vi "Cleanup.vi"(8 "error in":errorcluster, 11 "Refnum In":refnum<vi>) -> (0 "error out":errorcluster, 3 "Refnum Out":refnum<vi>)   [LabVIEW 2020]
doc: "Initializes the library with a serial comport as the transport method"
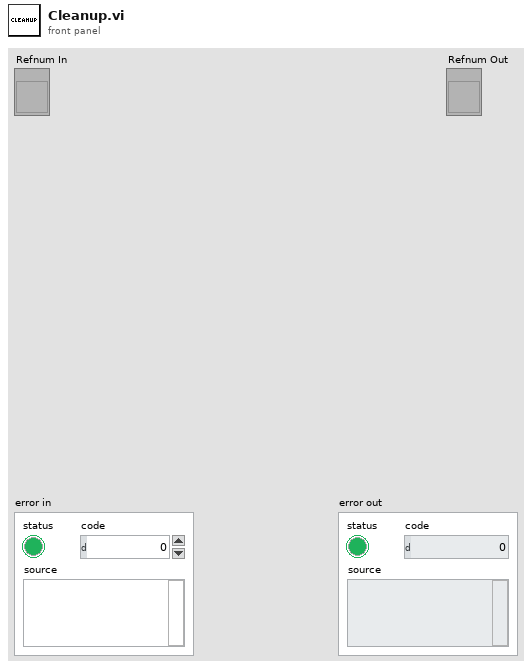
[diagram p1: front panel]
types:
  T1 = typedef "ConnectionParameters.ctl" = cluster{"Serial Communication":cluster{"Comport":refnum<visa-resource-name>, "No Response Timeout Ms":u32, "Response Complete Timeout Ms":u32, "Max Rx Length":u32, "Baud Rate":u32}, "Selected Transport":T2, "Initializer File Path":path, "Cleaner File Path":path, "Transporter File Path":path}
  T2 = typedef "SupportedTransports.ctl" = enum16{"Serial Communication Port"}
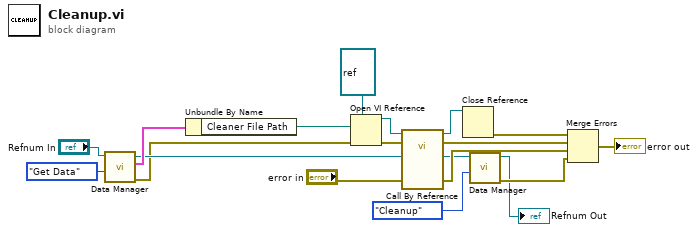
[diagram p0: block diagram]
diagram:
  n1 = call "Data Manager.vi"("Mode"=enum16{"Store Data", "Get Data", "Cleanup"}."Get Data", "Refnum In"="Refnum In") -> ("error out"=w7:errorcluster, "Data Out"=w11:T1, "Refnum Out"=w10:refnum<vi>)  [unwired: 7 in]
  n2 = Unbundle By Name(w11) -> ("Cleaner File Path"=w12:path)
  n3 = Open VI Reference(type specifier VI Refnum (for type only)=refnum<vi> refnum, vi path=w12, error in (no error)=w7) -> (vi reference=w17:refnum<vi>, error out=w18:errorcluster)  [unwired: 3 in]
  n4 = call-by-ref "?"(reference=w17, error in=w18, "error in"="error in", "Refnum In"=w10) -> (reference out=w16:refnum<vi>, error out=w15:errorcluster, 0:"error out"=w13:errorcluster, "Refnum Out"=w5:refnum<vi>)  [unwired: 8 in]
  n5 = Close Reference(reference=w16) -> (error out=w14:errorcluster)  [unwired: 1 in]
  n6 = call "Data Manager.vi"("Mode"=enum16{"Store Data", "Get Data", "Cleanup"}."Cleanup", "Refnum In"=w5) -> ("error out"=w4:errorcluster, "Refnum Out"=→"Refnum Out":refnum<vi>)  [unwired: 7 in, 1 out]
  n7 = Merge Errors(w14, w15, w13, w4) -> (→"error out":errorcluster)
